vi "Process_Table.vi"(7 "Type":T4 scale=0.0..2.0, 8 "error in (no error)":errorcluster, 10 "UI Data in":T1 {"Display"."Coffee" scale=0.0..80.0; "Display"."Chamber" scale=0.0..80.0; "Controls"."Type" scale=0.0..2.0; "Simulators"."Milk Level" min=0.0 max=100.0 step=10.0 scale=0.0..100.0 scale format="%#_3g"; "Simulators"."Bean Level" min=0.0 max=100.0 step=10.0 scale=0.0..100.0 scale format="%#_3g"; "Simulators"."Water Level" min=0.0 max=100.0 step=10.0 scale=0.0..100.0 scale format="%#_3g"}, 11 "System Status":T6) -> (0 "error out":errorcluster, 2 "UI Data out":T1 {"Display"."Coffee" scale=0.0..80.0; "Display"."Chamber" scale=0.0..80.0; "Controls"."Type" scale=0.0..2.0; "Simulators"."Milk Level" min=0.0 max=100.0 step=10.0 scale=0.0..100.0 scale format="%#_3g"; "Simulators"."Bean Level" min=0.0 max=100.0 step=10.0 scale=0.0..100.0 scale format="%#_3g"; "Simulators"."Water Level" min=0.0 max=100.0 step=10.0 scale=0.0..100.0 scale format="%#_3g"})   [LabVIEW 2026]
uses:
  controls/Type_Enum.ctl
  controls/System_Status.ctl
  controls/UI Data.ctl
  controls/Simulators.ctl
  controls/Controls.ctl
  controls/Display.ctl
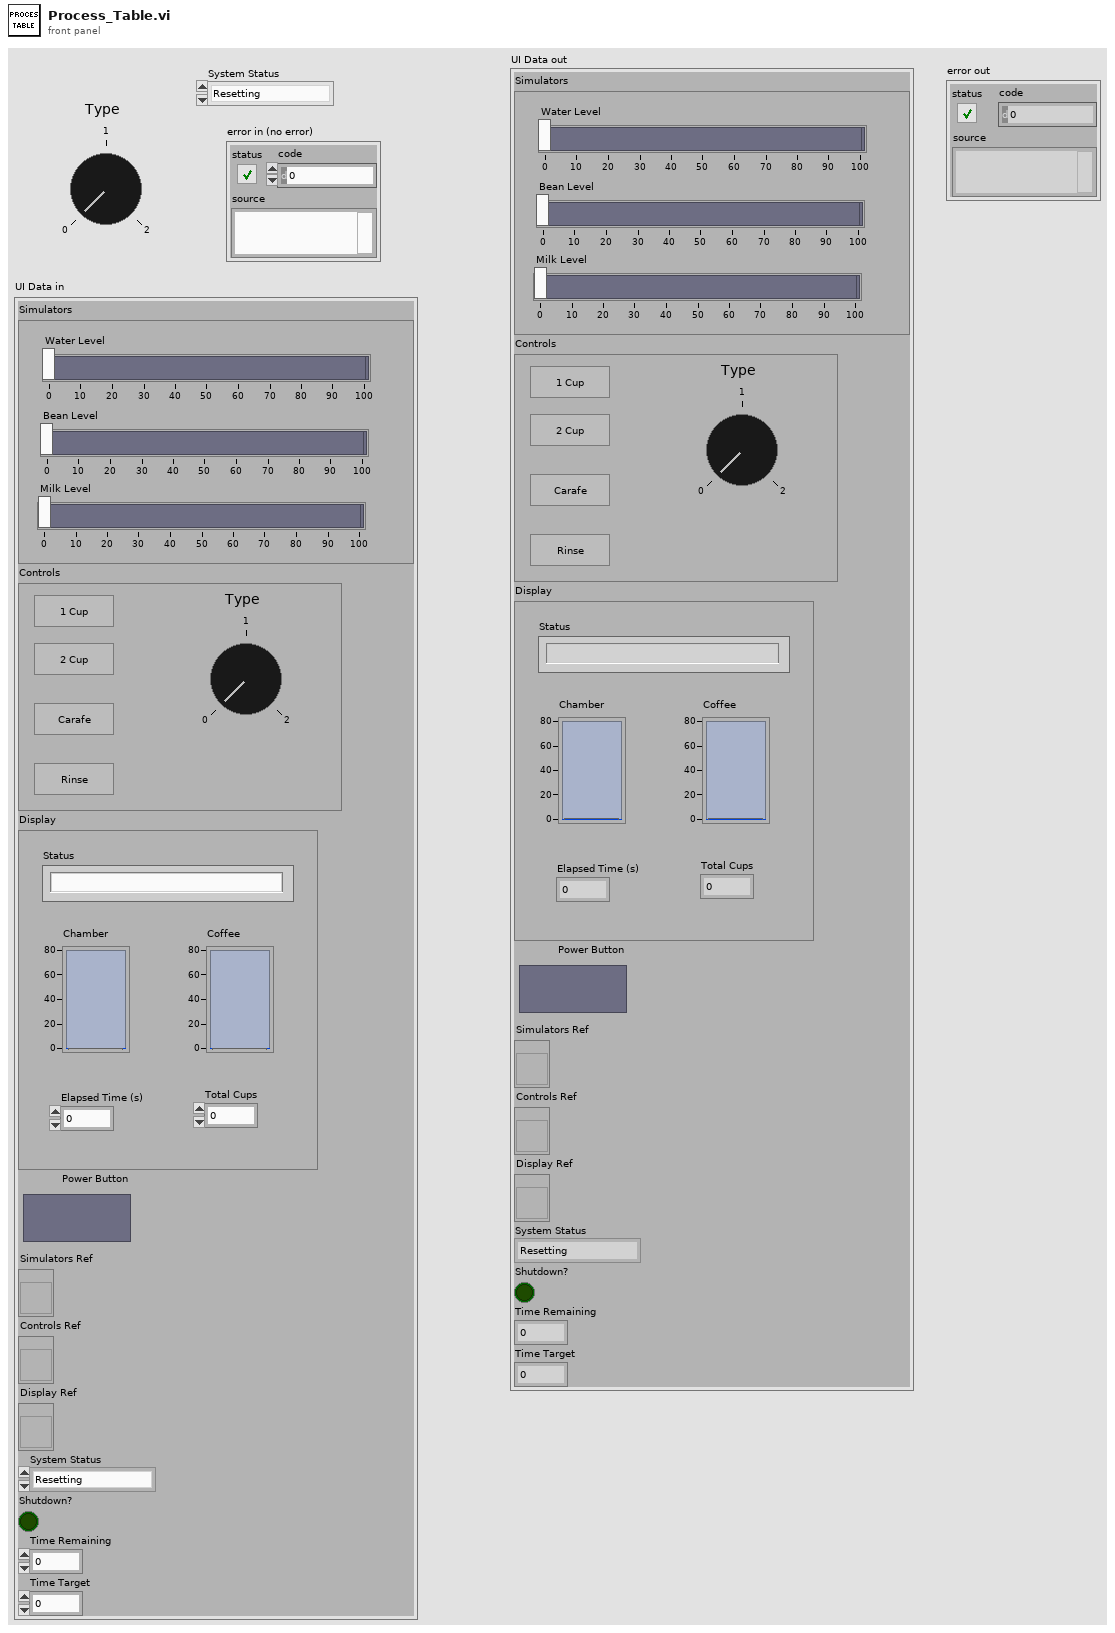
[diagram p1: front panel]
types:
  T1 = typedef "UI Data.ctl" = cluster{"Simulators":T2, "Controls":T3, "Display":T5, "Power Button":bool, "Simulators Ref":refnum<vi>, "Controls Ref":refnum<vi>, "Display Ref":refnum<vi>, "System Status":T6, "Shutdown?":bool, "Time Remaining":dbl, "Time Target":dbl}
  T2 = typedef "Simulators.ctl" = cluster{"Water Level":dbl, "Bean Level":dbl, "Milk Level":dbl}
  T3 = typedef "Controls.ctl" = cluster{"1 Cup":bool, "2 Cup":bool, "Carafe":bool, "Rinse":bool, "Type":T4}
  T4 = typedef "Type_Enum.ctl" = i16
  T5 = typedef "Display.ctl" = cluster{"Status":string, "Chamber":dbl, "Coffee":dbl, "Elapsed Time (s)":dbl, "Total Cups":dbl}
  T6 = typedef "System_Status.ctl" = enum16{"Resetting", "Heating Up", "Rinsing", "Threshold Check", "Ready for Brewing", "Grinding", "Brewing", "Dispensing", "Stepping", "Fulfilling", "Shutting Down"}
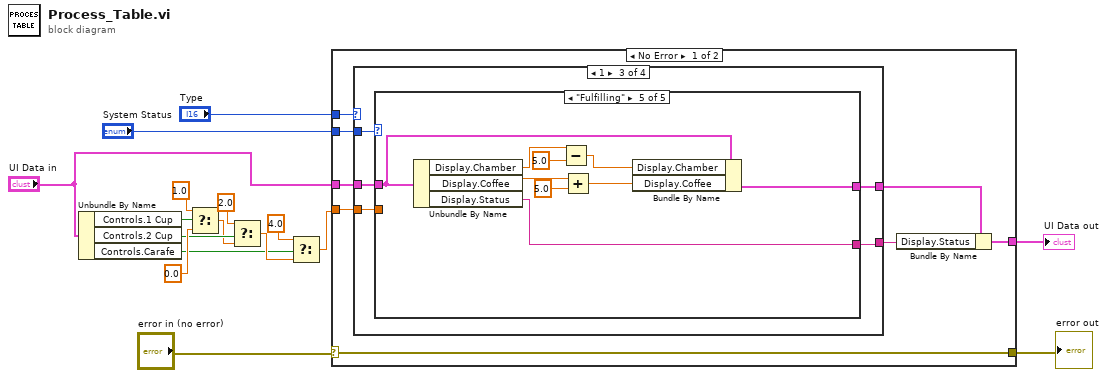
[diagram p0: block diagram]
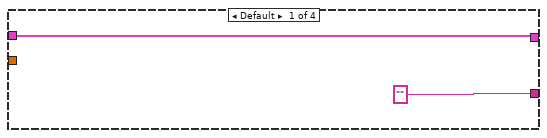
[diagram p2: hidden frame]
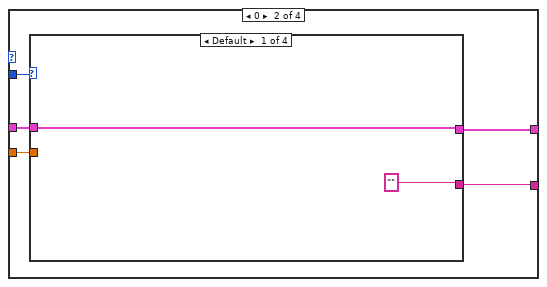
[diagram p3: hidden frame]
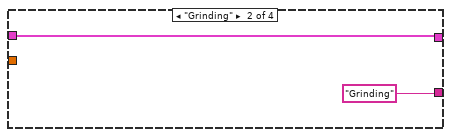
[diagram p4: hidden frame]
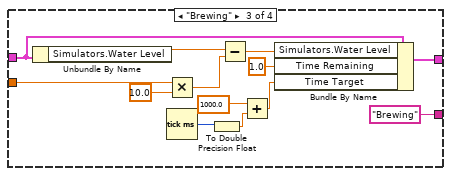
[diagram p5: hidden frame]
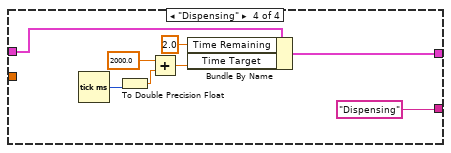
[diagram p6: hidden frame]
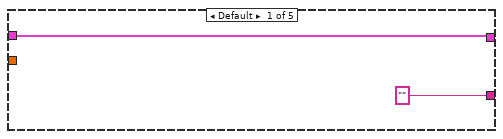
[diagram p7: hidden frame]
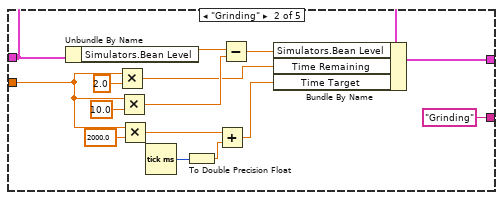
[diagram p8: hidden frame]
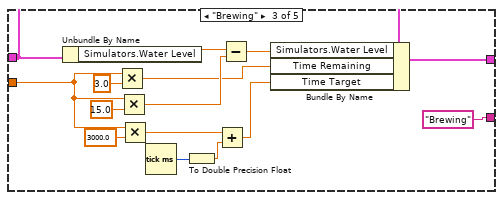
[diagram p9: hidden frame]
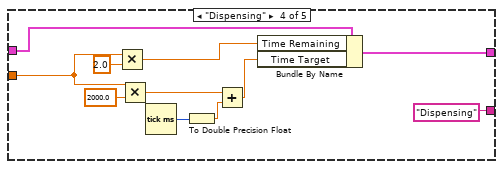
[diagram p10: hidden frame]
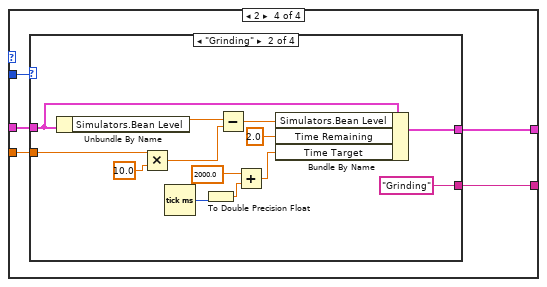
[diagram p11: hidden frame]
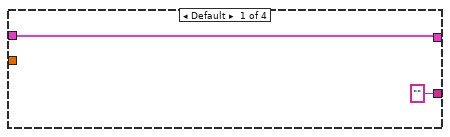
[diagram p12: hidden frame]
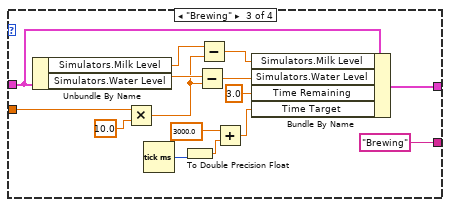
[diagram p13: hidden frame]
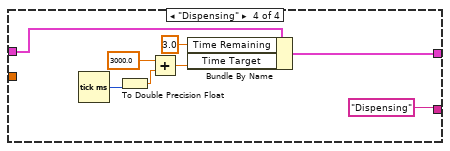
[diagram p14: hidden frame]
diagram:
  n1 = Unbundle By Name("UI Data in") -> ("Controls.1 Cup"=w11:bool, "Controls.2 Cup"=w8:bool, "Controls.Carafe"=w3:bool)
  n2 = Select(t=1.0, s=w11, f=0.0 ("t")) -> (s? t:f=w7:dbl)
  n3 = Select(t=2.0, s=w8, f=w7) -> (s? t:f=w5:dbl)
  n4 = Select(t=4.0, s=w3, f=w5) -> (s? t:f=w2:dbl)
  n5 = case shown="No Error" "error in (no error)" {
    selector: "error in (no error)" -> [w21 w158]
    tunnel: "Type" -> [w24 _]
    tunnel: "System Status" -> [w23 _]
    tunnel: "UI Data in" -> [w22 w157]
    tunnel: [w21 w158] -> w13
    tunnel: w2 -> [w20 _]
    tunnel: [w17 w157] -> w1
    frame No Error {
      n6 = case shown="1" w24 {
        tunnel: w23 -> [_ w31 w61 w118]
        tunnel: w22 -> [w26 w30 w60 w117]
        tunnel: [w26 w29 w59 w116] -> w19
        tunnel: w20 -> [_ w28 w58 w115]
        tunnel: ["" w27 w57 w114] -> w18
        frame Default {
        }
        frame 0 {
          n7 = case shown="Default" w31 {
            tunnel: w30 -> [w33 w35 w37 w53]
            tunnel: [w33 w35 w47 w54] -> w29
            tunnel: w28 -> [_ _ w40 _]
            tunnel: ["" "Grinding" "Brewing" "Dispensing"] -> w27
            frame Default {
            }
            frame "Grinding" {
            }
            frame "Brewing" {
              n8 = Unbundle By Name(w37) -> ("Simulators.Water Level"=w48:dbl)
              n9 = Multiply(x=w40, y=10.0) -> (x*y=w38:dbl)
              n10 = Tick Count (ms)() -> (millisecond timer value=w45:u32)
              n11 = To Double Precision Float(number=w45) -> (double precision float=w44:dbl)
              n12 = Subtract(x=w48, y=w38) -> (x-y=w46:dbl)
              n13 = Add(x=1000.0 ("y"), y=w44) -> (x+y=w42:dbl)
              n14 = Bundle By Name(cluster=w37, "Simulators.Water Level"=w46, "Time Remaining"=1.0, "Time Target"=w42) -> (w47:T1)
            }
            frame "Dispensing" {
              n15 = Tick Count (ms)() -> (millisecond timer value=w56:u32)
              n16 = To Double Precision Float(number=w56) -> (double precision float=w55:dbl)
              n17 = Add(x=2000.0 ("y"), y=w55) -> (x+y=w52:dbl)
              n18 = Bundle By Name(cluster=w53, "Time Remaining"=2.0, "Time Target"=w52) -> (w54:T1)
            }
          }
        }
        frame 1 {
          n19 = case shown="\"Fulfilling\"" w61 {
            tunnel: w60 -> [w63 w76 w91 w94 w111]
            tunnel: [w63 w77 w92 w104 w112] -> w59
            tunnel: w58 -> [_ w65 w80 w96 _]
            tunnel: ["" "Grinding" "Brewing" "Dispensing" w108] -> w57
            frame Default {
            }
            frame "Grinding" {
              n20 = Unbundle By Name(w76) -> ("Simulators.Bean Level"=w78:dbl)
              n21 = Multiply(x=w65, y=2.0 ("Time Remaining")) -> (x*y=w64:dbl)
              n22 = Multiply(x=w65, y=10.0) -> (x*y=w70:dbl)
              n23 = Multiply(x=w65, y=2000.0) -> (x*y=w68:dbl)
              n24 = Tick Count (ms)() -> (millisecond timer value=w74:u32)
              n25 = To Double Precision Float(number=w74) -> (double precision float=w73:dbl)
              n26 = Add(x=w68, y=w73) -> (x+y=w72:dbl)
              n27 = Subtract(x=w78, y=w70) -> (x-y=w75:dbl)
              n28 = Bundle By Name(cluster=w76, "Simulators.Bean Level"=w75, "Time Remaining"=w64, "Time Target"=w72) -> (w77:T1)
            }
            frame "Brewing" {
              n29 = Unbundle By Name(w91) -> ("Simulators.Water Level"=w93:dbl)
              n30 = Multiply(x=w80, y=3.0 ("Time Remaining")) -> (x*y=w79:dbl)
              n31 = Multiply(x=w80, y=15.0) -> (x*y=w85:dbl)
              n32 = Multiply(x=w80, y=3000.0) -> (x*y=w83:dbl)
              n33 = Tick Count (ms)() -> (millisecond timer value=w89:u32)
              n34 = To Double Precision Float(number=w89) -> (double precision float=w88:dbl)
              n35 = Add(x=w83, y=w88) -> (x+y=w87:dbl)
              n36 = Subtract(x=w93, y=w85) -> (x-y=w90:dbl)
              n37 = Bundle By Name(cluster=w91, "Simulators.Water Level"=w90, "Time Remaining"=w79, "Time Target"=w87) -> (w92:T1)
            }
            frame "Dispensing" {
              n38 = Multiply(x=w96, y=2.0 ("Time Remaining")) -> (x*y=w95:dbl)
              n39 = Multiply(x=w96, y=2000.0) -> (x*y=w99:dbl)
              n40 = Tick Count (ms)() -> (millisecond timer value=w103:u32)
              n41 = To Double Precision Float(number=w103) -> (double precision float=w102:dbl)
              n42 = Add(x=w99, y=w102) -> (x+y=w101:dbl)
              n43 = Bundle By Name(cluster=w94, "Time Remaining"=w95, "Time Target"=w101) -> (w104:T1)
            }
            frame "Fulfilling" {
              n44 = Unbundle By Name(w111) -> ("Display.Chamber"=w106:dbl, "Display.Coffee"=w113:dbl, "Display.Status"=w108:string)
              n45 = Subtract(x=w106, y=5.0) -> (x-y=w105:dbl)
              n46 = Add(x=w113, y=5.0) -> (x+y=w110:dbl)
              n47 = Bundle By Name(cluster=w111, "Display.Chamber"=w105, "Display.Coffee"=w110) -> (w112:T1)
            }
          }
        }
        frame 2 {
          n48 = case shown="\"Grinding\"" w118 {
            tunnel: w117 -> [w120 w131 w146 w153]
            tunnel: [w120 w132 w147 w154] -> w116
            tunnel: w115 -> [_ w123 w136 _]
            tunnel: ["" "Grinding" "Brewing" "Dispensing"] -> w114
            frame Default {
            }
            frame "Grinding" {
              n49 = Unbundle By Name(w131) -> ("Simulators.Bean Level"=w133:dbl)
              n50 = Multiply(x=w123, y=10.0) -> (x*y=w122:dbl)
              n51 = Tick Count (ms)() -> (millisecond timer value=w129:u32)
              n52 = To Double Precision Float(number=w129) -> (double precision float=w128:dbl)
              n53 = Subtract(x=w133, y=w122) -> (x-y=w130:dbl)
              n54 = Add(x=2000.0 ("y"), y=w128) -> (x+y=w126:dbl)
              n55 = Bundle By Name(cluster=w131, "Simulators.Bean Level"=w130, "Time Remaining"=2.0, "Time Target"=w126) -> (w132:T1)
            }
            frame "Brewing" {
              n56 = Unbundle By Name(w146) -> ("Simulators.Milk Level"=w139:dbl, "Simulators.Water Level"=w148:dbl)
              n57 = Multiply(x=w136, y=10.0) -> (x*y=w135:dbl)
              n58 = Tick Count (ms)() -> (millisecond timer value=w144:u32)
              n59 = To Double Precision Float(number=w144) -> (double precision float=w143:dbl)
              n60 = Subtract(x=w148, y=w135) -> (x-y=w145:dbl)
              n61 = Subtract(x=w139, y=w135) -> (x-y=w138:dbl)
              n62 = Add(x=3000.0 ("y"), y=w143) -> (x+y=w141:dbl)
              n63 = Bundle By Name(cluster=w146, "Simulators.Milk Level"=w138, "Simulators.Water Level"=w145, "Time Remaining"=3.0, "Time Target"=w141) -> (w147:T1)
            }
            frame "Dispensing" {
              n64 = Tick Count (ms)() -> (millisecond timer value=w156:u32)
              n65 = To Double Precision Float(number=w156) -> (double precision float=w155:dbl)
              n66 = Add(x=3000.0 ("y"), y=w155) -> (x+y=w152:dbl)
              n67 = Bundle By Name(cluster=w153, "Time Remaining"=3.0, "Time Target"=w152) -> (w154:T1)
            }
          }
        }
      }
      n68 = Bundle By Name(cluster=w19, "Display.Status"=w18) -> (w17:T1)
    }
    frame Error {
    }
  }
  "UI Data out" <- w1
  "error out" <- w13
